vi "CLFNCheckMatch.vi"(8 "error in (no error)":errorcluster) -> (0 "error out":errorcluster)   [LabVIEW 2020]
uses:
  <vilib>/Utility/traverseref.llb/TRef TravTarget.ctl
  <vilib>/Utility/traverseref.llb/VI Scripting - Traverse.lvlib
panel:
  out "dup file":path
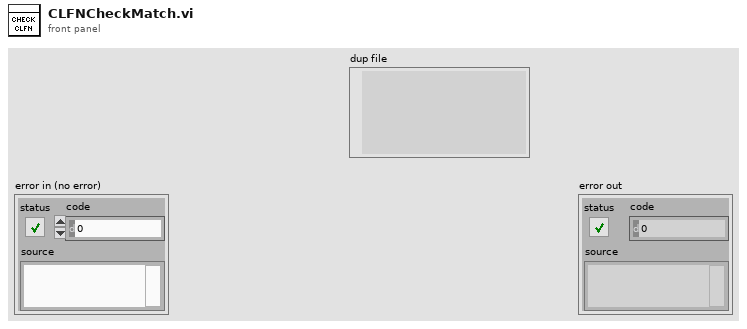
[diagram p1: front panel]
types:
  T1 = typedef "TRef TravTarget.ctl" = enum16{"FP", "BD", "Other"}
  T2 = enum32{"Invalid", "Standard", "Closed", "Hidden", "Minimized", "Maximized"}
  T3 = cluster{"Parameter Name":string, "Num Dimensions":i32, "Parameter Type":enum16{"Numeric", "Array", "String", "Waveform", "Digital Waveform", "Digital Table", "ActiveX", "Any", "Instance Data Pointer", "Void"}, "Numeric Type":enum16{"I8", "I16", "I32", "I64", "U8", "U16", "U32", "U64", "SGL", "DBL", "PTR INT", "PTR UINT"}, "Param Passing":enum16{"By Value", "Pointer To Value"}, "Array Passing":enum16{"Array Data Pointer", "Array Handle", "Array Handle Pointer"}, "String Passing":enum16{"C String Pointer", "Pascal String Pointer", "String Handle", "String Handle Pointer"}, "Adapt Format":enum16{"By Value", "Pointer To Value"}, "ActiveX Types":enum16{"ActiveX Variant Pointer", "IDispatch* Pointer", "IUnknown* Pointer"}, "Const (unused)":bool, "Minimum Size":string}[]
  T4 = cluster{"FuncName":string, "ParamInfo":cluster{"Parameter Name":string, "Num Dimensions":i32, "Parameter Type":enum16{"Numeric", "Array", "String", "Waveform", "Digital Waveform", "Digital Table", "ActiveX", "Any", "Instance Data Pointer", "Void"}, "Numeric Type":enum16{"I8", "I16", "I32", "I64", "U8", "U16", "U32", "U64", "SGL", "DBL", "PTR INT", "PTR UINT"}, "Param Passing":enum16{"By Value", "Pointer To Value"}, "Array Passing":enum16{"Array Data Pointer", "Array Handle", "Array Handle Pointer"}, "String Passing":enum16{"C String Pointer", "Pascal String Pointer", "String Handle", "String Handle Pointer"}, "Adapt Format":enum16{"By Value", "Pointer To Value"}, "ActiveX Types":enum16{"ActiveX Variant Pointer", "IDispatch* Pointer", "IUnknown* Pointer"}, "Const (unused)":bool, "Minimum Size":string}[]}
  T5 = typedef "LVPositionTypeDef.ctl" = cluster{"Left":i32, "Top":i32}
  T6 = cluster{"Parameter Name":string, "Num Dimensions":i32, "Parameter Type":enum16{"Numeric", "Array", "String", "Waveform", "Digital Waveform", "Digital Table", "ActiveX", "Any", "Instance Data Pointer", "Void"}, "Numeric Type":enum16{"I8", "I16", "I32", "I64", "U8", "U16", "U32", "U64", "SGL", "DBL", "PTR INT", "PTR UINT"}, "Param Passing":enum16{"By Value", "Pointer To Value"}, "Array Passing":enum16{"Array Data Pointer", "Array Handle", "Array Handle Pointer"}, "String Passing":enum16{"C String Pointer", "Pascal String Pointer", "String Handle", "String Handle Pointer"}, "Adapt Format":enum16{"By Value", "Pointer To Value"}, "ActiveX Types":enum16{"ActiveX Variant Pointer", "IDispatch* Pointer", "IUnknown* Pointer"}, "Const (unused)":bool, "Minimum Size":string}
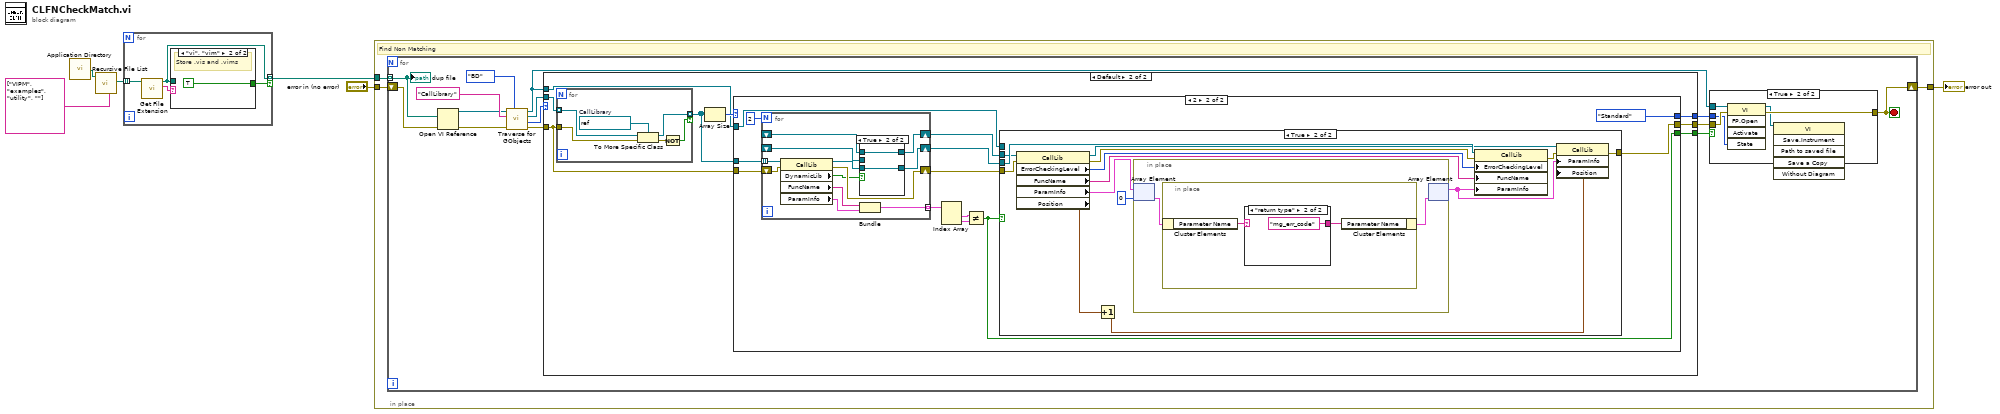
[diagram p0: block diagram]
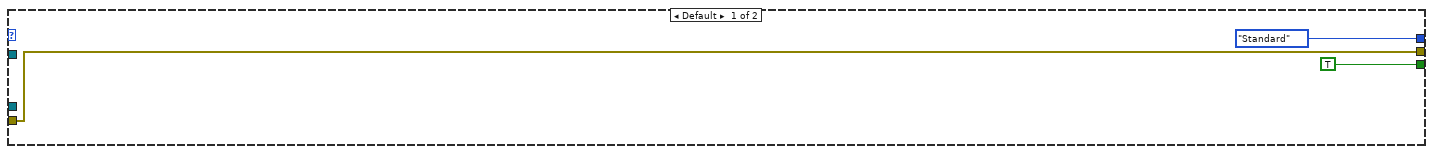
[diagram p5: hidden frame]
diagram:
  n1 = call <vilib>:"Application Directory.vi"() -> ("Application Directory"=w2:path)
  n2 = call <vilib>:"Recursive File List.vi"("Folders to Exclude"=string[] ["VIPM", "examples", "utility", ""], "Folder Path"=w2) -> ("All Files in Dir"=w1:path[])  [unwired: 5 in, 4 out]
  n3 = for {
    tunnel: w1 -> [w10] mode=indexing
    tunnel: [w7] -> w6 mode=indexing if=w8
    n4 = call <vilib>:"Get File Extension.vi"("file"=w10) -> ("lowercase file extension"=w9:string, "dup file"=w7:path)  [unwired: 6 in, 3 out]
    n5 = case shown="\"vi\", \"vim\"" w9 {
      tunnel: [_ TRUE] -> w8
      tunnel: w7 -> [_ _]
      frame Default {
      }
      frame "vi", "vim" {
        # "Store .vis and .vims"
      }
    }
  }
  n6 = in-place {
    in-place-border: [w12] -> w5
    in-place-border: w6 -> [w14]
    in-place-border: "error in (no error)" -> [w13]
    # "Find Non Matching"
    n7 = for {
      tunnel: w14 -> [w28] mode=indexing
      shift-right: [w17] -> w12
      shift-left: w13 -> [w27]
      stop <- w17 stop-if-true
      n8 = Open VI Reference(vi path=w28, error in (no error)=w27) -> (vi reference=w23:refnum<vi>, error out=w22:errorcluster)  [unwired: 4 in]
      n9 = call <vilib>:"Traverse for GObjects.vi"("Traverse Target"=TRef_TravTarget."BD", "error in (no error)"=w22, "Class Name"="CallLibrary", "VI Refnum"=w23) -> ("error out"=w26:errorcluster, "# of Refs"=w20:i32, "References"=w21:refnum<vi>[], "dup VI Refnum"=w15:refnum<vi>)  [unwired: 4 in]
      n10 = case shown="Default" w20 {
        tunnel: [w35 w41] -> w18
        tunnel: w26 -> [w35 w42]
        tunnel: w21 -> [_ w43]
        tunnel: [_ w38] -> w19
        tunnel: [_ w37] -> w16
        tunnel: w15 -> [_ w36]
        frame 0 {
        }
        frame Default {
          n11 = for {
            tunnel: w42 -> [w102]
            tunnel: w43 -> [w100] mode=indexing
            tunnel: [w98] -> w40 mode=indexing if=w97
            w101 = refnum<vi> refnum  # CallLibrary
            n12 = To More Specific Class(target class=w101, reference=w100, error in=w102) -> (specific class reference=w98:refnum<vi>, error out=w99:errorcluster)
            n13 = Not(x=w99) -> (.not. x?=w97:bool)
          }
          n14 = Array Size(array=w40) -> (size(s)=w39:i32)
          n15 = case shown="2" w39 {
            tunnel: w42 -> [w46 w59]
            tunnel: [w46 w53] -> w41
            tunnel: w40 -> [_ w58]
            tunnel: [TRUE w49] -> w38
            tunnel: [T2."Standard" ("State") T2."Standard" ("State")] -> w37
            tunnel: w36 -> [_ w50]
            frame Default {
            }
            frame 2 {
              n16 = for {
                N: 2 -> [_]
                shift-right: [w92] -> w54
                shift-left: w59 -> [w90]
                tunnel: w58 -> [w91] mode=indexing
                shift-right: [w87] -> w56
                shift-left: _ -> [w86]
                shift-right: [w85] -> w55
                shift-left: _ -> [w84]
                tunnel: [w81] -> w57 mode=indexing
                n17 = property class="CallLib"(reference=w91, error in=w90) -> (reference out=w88:refnum<vi>, error out=w92:errorcluster, "DynamicLib"=w89:bool, "FuncName"=w83:string, "ParamInfo"=w82:T3)
                n18 = case shown="True" w89 {
                  tunnel: w88 -> [w94 w96]
                  tunnel: [w93 w96] -> w87
                  tunnel: w86 -> [w93 _]
                  tunnel: [w94 w95] -> w85
                  tunnel: w84 -> [_ w95]
                  frame False {
                  }
                  frame True {
                  }
                }
                n19 = Bundle("FuncName"=w83, "ParamInfo"=w82) -> (w81:T4)  [unwired: 1 in]
              }
              n20 = Index Array(array=w57) -> (element #1=w48:T4, element #2=w47:T4)  [unwired: 2 in]
              n21 = Not Equal?(x=w48, y=w47) -> (x != y?=w49:bool)
              n22 = case shown="True" w49 {
                tunnel: w56 -> [_ w74]
                tunnel: w55 -> [_ w73]
                tunnel: w54 -> [w60 w70]
                tunnel: [w60 w66] -> w53
                tunnel: w50 -> [_ _]
                frame False {
                }
                frame True {
                  n23 = property class="CallLib"(reference=w73, error in=w70) -> (reference out=w65:refnum<vi>, error out=w69:errorcluster, "ErrorCheckingLevel"=w72:u32, "FuncName"=w71:string, "ParamInfo"=w68:T3, "Position"=w62:T5)
                  n24 = Increment(x=w62) -> (x+1=w61:T5)
                  n25 = in-place {
                    n26 = in-place-array #1(w68, 0) -> (w76:T6)
                    n27 = in-place {
                      n28 = in-place-cluster #2(w76) -> ("Parameter Name"=w78:string)
                      n29 = case shown="\"return type\"" w78 {
                        selector: w78 -> [w79 _]
                        tunnel: [w79 "mg_err_code"] -> w77
                        frame Default {
                        }
                        frame "return type" {
                        }
                      }
                      n30 = in-place-cluster #2("Parameter Name"=w77) -> (w75:T6)
                    }
                    n31 = in-place-array #1(w75) -> (w64:T3)  [unwired: 1 out]
                  }
                  n32 = property class="CallLib"(reference=w74, error in=w69, "ErrorCheckingLevel"=w72, "FuncName"=w71, "ParamInfo"=w64) -> (error out=w67:errorcluster)  [unwired: 1 out]
                  n33 = property class="CallLib"(reference=w65, error in=w67, "ParamInfo"=w64, "Position"=w61) -> (error out=w66:errorcluster)  [unwired: 1 out]
                }
              }
            }
          }
        }
      }
      n34 = case shown="True" w19 {
        tunnel: w15 -> [_ w34]
        tunnel: w18 -> [w29 w33]
        tunnel: [w29 w32] -> w17
        tunnel: w16 -> [_ w31]
        frame False {
        }
        frame True {
          n35 = invoke class="VI" method="FP.Open"(reference=w34, error in=w33, "State"=w31) -> (reference out=w30:refnum<vi>, error out=w32:errorcluster)  [unwired: 2 in, 3 out]
          n36 = invoke class="VI" method="Save.Instrument"(reference=w30) -> ()  [unwired: 5 in, 6 out]
        }
      }
      "dup file" <- w28
    }
  }
  "error out" <- w5
